vi "S1_parametetsSetting2017.vi"() -> ()   [LabVIEW 2012]
uses:
  2015myGlobal 1.vi
panel:
  in  "停留時間(秒)":dbl=4.0
  in  "stop":bool
  in  "重複次數":i32=5
  in  "上升時間(秒)":dbl=4.0
  out "馬達速度\n設定參數":i32
  out "前進Steps":i32
  in  "前進距離(mm)":dbl=4.0
  # "距離"
  # "前\n進\n距\n離\n(mm)"
  # "停留時間(秒)"
  # "上升時間(秒)"
  # "時間"
  # "停留時間(秒)"
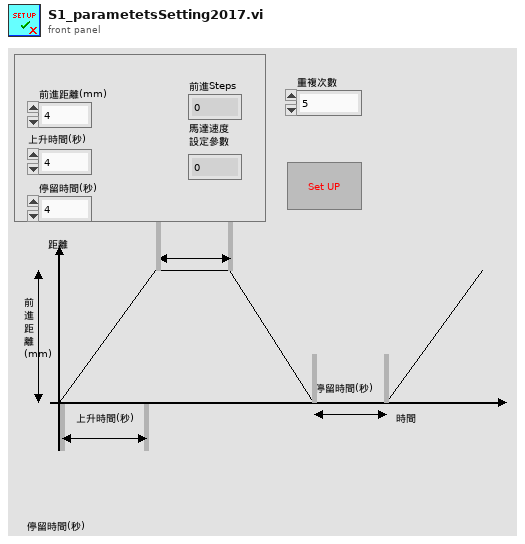
[diagram p1: front panel]
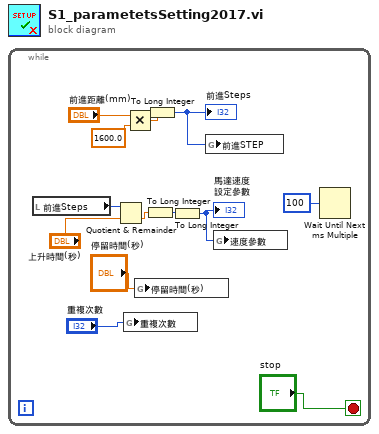
[diagram p0: block diagram]
diagram:
  n1 = while {
    stop <- "stop" stop-if-true
    n2 = local read "前進Steps"() -> (w8:i32)
    n3 = Quotient & Remainder(x=w8, y="上升時間(秒)") -> (floor(x/y)=w6:dbl)  [unwired: 1 out]
    n4 = global write "2015myGlobal 1.vi" "重複次數"("重複次數") -> ()
    n5 = Multiply(x="前進距離(mm)", y=1600.0) -> (x*y=w11:dbl)
    n6 = global write "2015myGlobal 1.vi" "停留時間(秒)"("停留時間(秒)") -> ()
    n7 = To Long Integer(number=w6) -> (32bit integer=w5:i32)
    n8 = To Long Integer(number=w11) -> (32bit integer=w10:i32)
    "前進Steps" <- w10
    n9 = To Long Integer(number=w5) -> (32bit integer=w9:i32)
    "馬達速度\n設定參數" <- w9
    n10 = global write "2015myGlobal 1.vi" "前進STEP"(w10) -> ()
    n11 = global write "2015myGlobal 1.vi" "速度參數"(w9) -> ()
    n12 = Wait Until Next ms Multiple(millisecond multiple=u32 100) -> ()  [unwired: 1 out]
  }
